vi "GoPro Set Power.vi"(10 "On?":bool, 11 "Gopro DevRef":T1) -> (3 "Output DevRef":T1)   [LabVIEW 2015]
uses:
  GoPro DevRef.ctl
  <vilib>/httpClient/ClientHandle.ctl
  GET Parameter.ctl
  <vilib>/httpClient/LabVIEWHTTPClient.lvlib
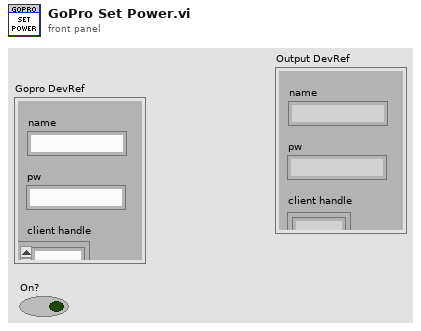
[diagram p1: front panel]
types:
  T1 = typedef "GoPro DevRef.ctl" = cluster{"name":string, "pw":string, "client handle":T2}
  T2 = typedef "LabVIEWHTTPClient.lvlib/ClientHandle.ctl" = refnum<k1>
  T3 = typedef "GET Parameter.ctl" = cluster{"key":string, "val":string}
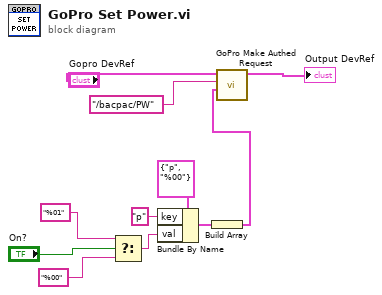
[diagram p0: block diagram]
diagram:
  n1 = Select(t="%01" ("key"), s="On?", f="%00" ("key")) -> (s? t:f=w5:string)
  n2 = Bundle By Name(cluster=T3 {"key"="p", "val"="%00"} ("element"), "key"="p", "val"=w5) -> (w9:T3)
  n3 = Build Array(w9) -> (w10:T3[])
  n4 = call "GoPro Make Authed Request.vi"("Params"=w10, "url"="/bacpac/PW", "Gopro DevRef"="Gopro DevRef") -> ("Output DevRef"=→"Output DevRef":T1)  [unwired: 5 in, 3 out]
